vi "DigitalAQ Puerto.vi"(8 "error in":errorcluster, 11 "DAQmx Board Name":tag="DAQSim1") -> (0 "error out":errorcluster, 3 "Classic DAQmx Task Name":refnum<k21>)   [LabVIEW 2020]
uses:
  <vilib>/DAQmx/create/channels.llb/DAQmx Create Channel (DI-Digital Input).vi
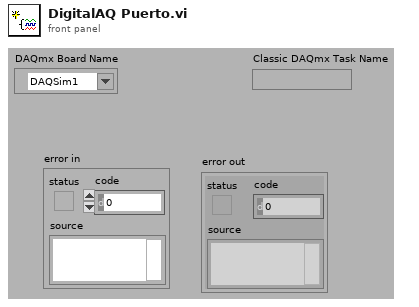
[diagram p1: front panel]
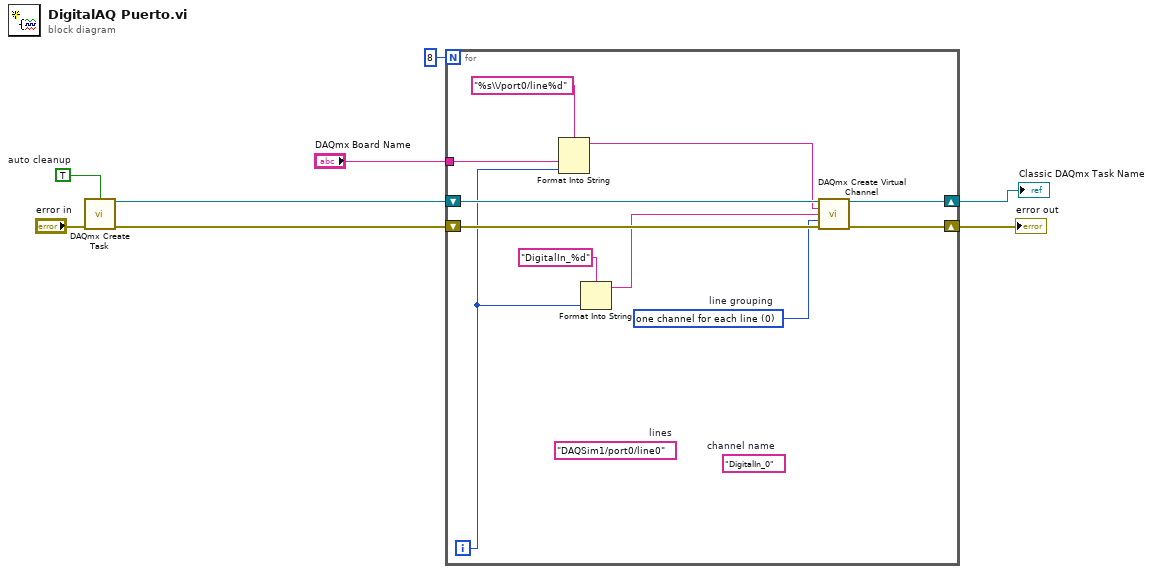
[diagram p0: block diagram]
diagram:
  w6 = TRUE  # auto cleanup
  n1 = call <vilib>:"DAQmx Create Task.vi"("auto cleanup"=w6, "error in"="error in") -> ("task out"=w5:refnum<k21>, "error out"=w7:errorcluster)  [unwired: 12 in]
  n2 = for {
    N: 8 -> [_]
    shift-right: [w16] -> w4
    shift-left: w7 -> [w19]
    shift-right: [w15] -> w1
    shift-left: w5 -> [w18]
    tunnel: "DAQmx Board Name" -> [w12]
    i -> [w11]
    w17 = 0 items=["one channel for each line", "one channel for all lines"]  # line grouping
    (unwired) "DigitalIn_0"  # channel name
    (unwired) "DAQSim1/port0/line0"  # lines
    n3 = Format Into String(format string="%s\\/port0/line%d", w12, w11) -> (resulting string=w9:string)  [unwired: 2 in, 1 out]
    n4 = Format Into String(format string="DigitalIn_%d", w11) -> (resulting string=w10:string)  [unwired: 2 in, 1 out]
    n5 = call-poly <vilib>:"DAQmx Create Virtual Channel.vi"("task in"=w18, "lines"=w9, "name to assign"=w10, "line grouping"=w17, "error in"=w19) -> ("task out"=w15:refnum<k21>, "error out"=w16:errorcluster)  [unwired: 9 in]
  }
  "error out" <- w4
  "Classic DAQmx Task Name" <- w1
